vi "Evaluta emibin top Header.vi"(7 "bin ID header":T1={"Fixed code"=255158202, "File type Std"=0, "File type ID"=1, "File type Version"=0} {"File type Std" format="%.0x"; "Fixed code" format="%.0x"; "File type ID" format="%.0x"; "File type Version" format="%.0x"}, 11 "error in (no error)":errorcluster) -> (3 "File complete ID":u32, 4 "Correct Hader":bool, 6 "File type Std":u8 format="%.0x", 8 "File type ID":u16=1 format="%.0x", 10 "File type Version":u8 format="%.0x", 15 "error out":errorcluster)   [LabVIEW 2011]
uses:
  Header.ctl
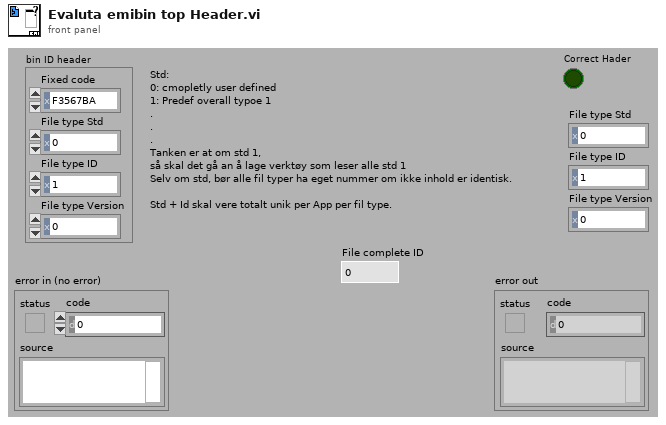
[diagram p1: front panel]
types:
  T1 = typedef "Header.ctl" = cluster{"Fixed code":u32, "File type Std":u8, "File type ID":u16, "File type Version":u8}
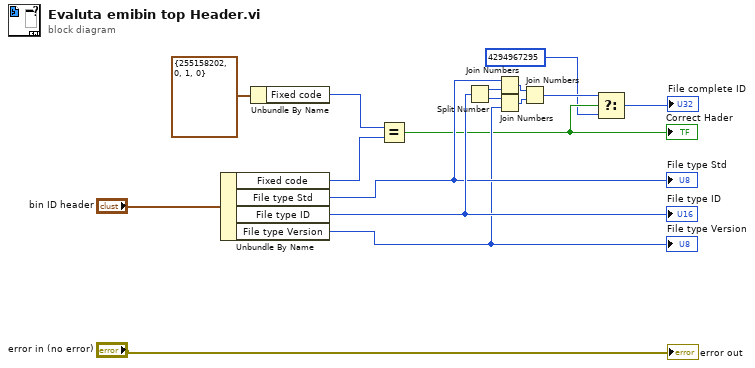
[diagram p0: block diagram]
diagram:
  n1 = Unbundle By Name("bin ID header") -> ("Fixed code"=w12:u32, "File type Std"=w8:u8, "File type ID"=w11:u16, "File type Version"=w7:u8)
  "File type Version" <- w7
  "File type ID" <- w11
  "File type Std" <- w8
  n2 = Unbundle By Name(T1 {"Fixed code"=255158202, "File type Std"=0, "File type ID"=1, "File type Version"=0} ("bin ID header")) -> ("Fixed code"=w13:u32)
  n3 = Equal?(x=w13, y=w12) -> (x = y?=w4:bool)
  "Correct Hader" <- w4
  n4 = Split Number(x=w11) -> (hi(x)=w10:u8, lo(x)=w9:u8)
  n5 = Join Numbers(hi=w8, lo=w10) -> ((hi.lo)=w6:u16)
  n6 = Join Numbers(hi=w9, lo=w7) -> ((hi.lo)=w5:u16)
  n7 = Join Numbers(hi=w6, lo=w5) -> ((hi.lo)=w3:u32)
  n8 = Select(t=w3, s=w4, f=u32 4294967295) -> (s? t:f=→"File complete ID":u32)
  "error out" <- "error in (no error)"
